vi "ABC Save Data.vi"(7 "Folder":path=path "C:/Amira Data/Strip", 8 "ErrIn":errorcluster, 11 "Data":dbl[][](array[numeric])) -> (0 "ErrOut":errorcluster)   [LabVIEW 2020]
uses:
  <vilib>/Utility/file.llb/Write Delimited Spreadsheet (string).vi
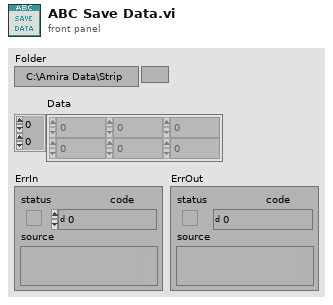
[diagram p1: front panel]
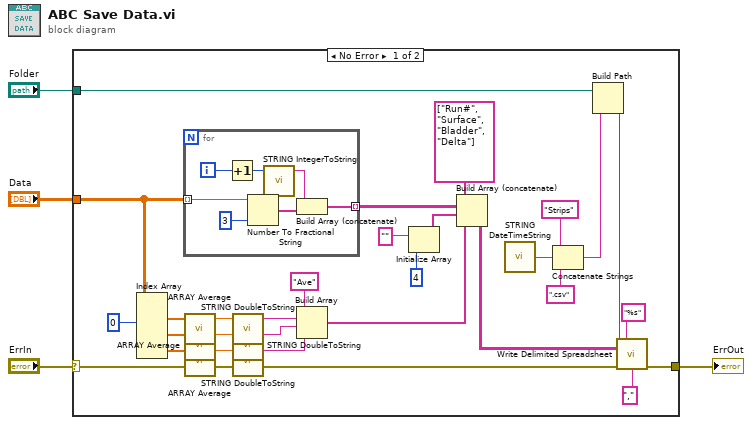
[diagram p0: block diagram]
diagram:
  n1 = case shown="No Error" "ErrIn" {
    selector: "ErrIn" -> [w5 w41]
    tunnel: "Folder" -> [w25 _]
    tunnel: [w24 w41] -> w3
    tunnel: "Data" -> [w20 _]
    frame No Error {
      n2 = Index Array(array=w20, index (col) #1=0 ("disabled index (col)")) -> (element #1=w18:dbl[], element #2=w17:dbl[], element #3=w16:dbl[])  [unwired: 5 in]
      n3 = for {
        tunnel: [w35] -> w26 mode=indexing
        tunnel: w20 -> [w38] mode=indexing
        i -> [w37]
        n4 = Increment(x=w37) -> (x+1=w36:i32)
        n5 = Number To Fractional String(number=w38, precision (6)=i16 3) -> (F-format string=w40:string[])  [unwired: 2 in]
        n6 = call <userlib>:"STRING IntegerToString.vi"("Num"=w36) -> ("IntStr"=w34:string)  [unwired: 4 in]
        n7 = Build Array (concatenate)(w34, w40) -> (w35:string[])
      }
      n8 = call <userlib>:"ARRAY Average.vi"("Array"=w18) -> ("Ave"=w15:dbl)  [unwired: 4 in]
      n9 = call <userlib>:"ARRAY Average.vi"("Array"=w17) -> ("Ave"=w14:dbl)  [unwired: 4 in]
      n10 = call <userlib>:"ARRAY Average.vi"("Array"=w16) -> ("Ave"=w13:dbl)  [unwired: 4 in]
      n11 = call <userlib>:"STRING DoubleToString.vi"("Num"=w15) -> ("DblStr"=w10:string)  [unwired: 3 in]
      n12 = call <userlib>:"STRING DoubleToString.vi"("Num"=w14) -> ("DblStr"=w11:string)  [unwired: 3 in]
      n13 = call <userlib>:"STRING DoubleToString.vi"("Num"=w13) -> ("DblStr"=w12:string)  [unwired: 3 in]
      n14 = Build Array("Ave" ("element"), w10, w11, w12) -> (w8:string[])
      n15 = Initialize Array("", 4 ("dimension size")) -> (w21:string[])
      n16 = Build Array (concatenate)(string[] ["Run#", "Surface", "Bladder", "Delta"], w26, w21, w8) -> (w28:string[][])
      n17 = call <userlib>:"STRING DateTimeString.vi"() -> ("DateTimeStr"=w30:string)  [unwired: 2 in]
      n18 = Concatenate Strings("Strips" ("string"), w30, ".csv" ("string")) -> (w32:string)
      n19 = Build Path(base path=w25, name or relative path=w32) -> (appended path=w33:path)
      n20 = call-poly <vilib>:"Write Delimited Spreadsheet.vi"("file path (dialog if empty)"=w33, "format (%s)"="%s", "2D data"=w28, "error in (no error)"=w5, "delimiter (\\t)"="," ("delimiter (\\t)")) -> ("error out"=w24:errorcluster)  [unwired: 9 in, 1 out]
    }
    frame Error {
    }
  }
  "ErrOut" <- w3
